vi "Find Analog Replay.vi"(8 "error in (no error)":errorcluster, 9 "RIO Device Address":string, 10 "Name":string, 11 "APU in":refnum<k24>) -> (0 "error out":errorcluster, 2 "Analog Replay":refnum<k24>, 3 "APU out":refnum<k24>)   [LabVIEW 2015, in "Engine Simulation Toolkit Scripting API.lvlib"]
uses:
  Engine Simulation Toolkit Scripting API.lvlib
  NationalInstruments.VeriStand.SystemDefinitionAPI
  Shared/Constants and GUIDs.vi
  Shared/Engine Simulation Toolkit Shared.lvlib
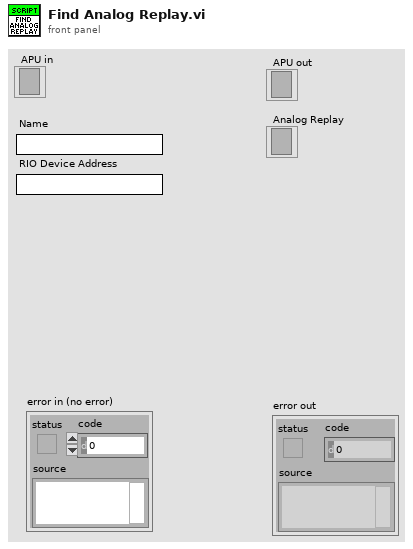
[diagram p1: front panel]
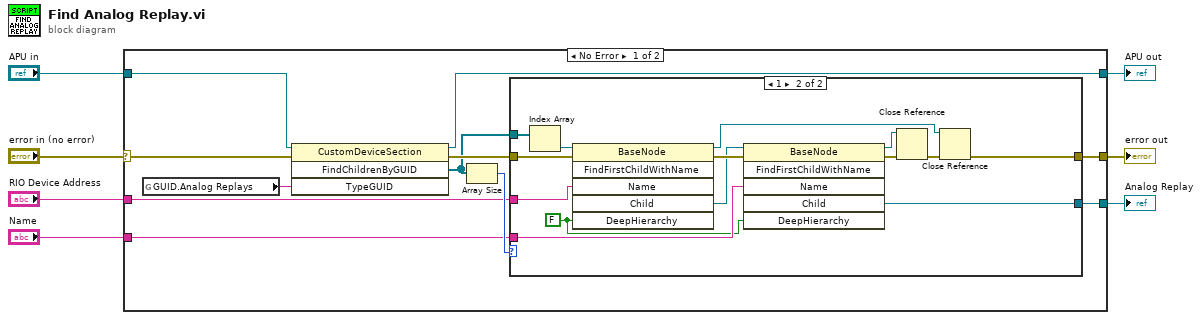
[diagram p0: block diagram]
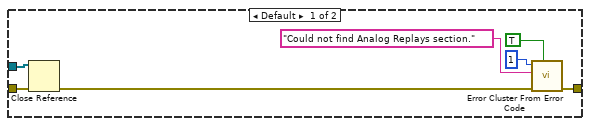
[diagram p2: hidden frame]
diagram:
  n1 = case shown="No Error" "error in (no error)" {
    selector: "error in (no error)" -> [w10 w41]
    tunnel: [w12 w41] -> w7
    tunnel: "APU in" -> [w18 w40]
    tunnel: [w11 w40] -> w4
    tunnel: "RIO Device Address" -> [w13 _]
    tunnel: "Name" -> [w9 _]
    tunnel: [w8 _] -> w1
    frame No Error {
      n2 = global read "Constants and GUIDs.vi" "GUID.Analog Replays"() -> (w17:string)
      n3 = invoke class="CustomDeviceSection" method="FindChildrenByGUID"(reference=w18, error in=w10, "TypeGUID"=w17) -> (reference out=w11:refnum<k24>, error out=w15:errorcluster, "FindChildrenByGUID"=w14:refnum<k24>[])  [unwired: 1 in, 1 out]
      n4 = Array Size(array=w14) -> (size(s)=w16:i32)
      n5 = case shown="1" w16 {
        tunnel: [w25 w29] -> w12
        tunnel: w15 -> [w20 w34]
        tunnel: w14 -> [w21 w39]
        tunnel: w13 -> [_ w37]
        tunnel: w9 -> [_ w28]
        tunnel: [_ w27] -> w8
        frame Default {
          n6 = Close Reference(reference=w21, error in (no error)=w20) -> (error out=w19:errorcluster)
          n7 = call <vilib>:"Error Cluster From Error Code.vi"("show call chain? (False)"=TRUE, "error in (no error)"=w19, "error message (\"\")"="Could not find Analog Replays section." ("error message (\"\")"), "error code (0)"=1) -> ("error out"=w25:errorcluster)  [unwired: 5 in]
        }
        frame 1 {
          w26 = FALSE ("DeepHierarchy")
          n8 = Index Array(array=w39) -> (element=w38:refnum<k24>)  [unwired: 1 in]
          n9 = invoke class="BaseNode" method="FindFirstChildWithName"(reference=w38, error in=w34, "Name"=w37, "DeepHierarchy"=w26) -> (reference out=w30:refnum<k24>, error out=w36:errorcluster, "Child"=w35:refnum<k24>)  [unwired: 2 in, 3 out]
          n10 = invoke class="BaseNode" method="FindFirstChildWithName"(reference=w35, error in=w36, "Name"=w28, "DeepHierarchy"=w26) -> (reference out=w33:refnum<k24>, error out=w32:errorcluster, "Child"=w27:refnum<k24>)  [unwired: 2 in, 3 out]
          n11 = Close Reference(reference=w33, error in (no error)=w32) -> (error out=w31:errorcluster)
          n12 = Close Reference(reference=w30, error in (no error)=w31) -> (error out=w29:errorcluster)
        }
      }
    }
    frame Error {
    }
  }
  "error out" <- w7
  "APU out" <- w4
  "Analog Replay" <- w1
